vi "Test.vi"() -> ()   [LabVIEW 2022 SP3]
panel:
  out "error IO":errorcluster
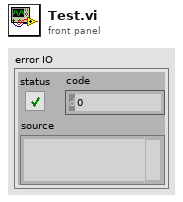
[diagram p1: front panel]
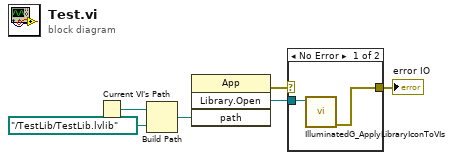
[diagram p0: block diagram]
diagram:
  n1 = Current VI's Path() -> (path=w5:path)
  n2 = Build Path(base path=w5, name or relative path=path "../TestLib/TestLib.lvlib") -> (appended path=w3:path)
  n3 = invoke class="App" method="Library.Open"("path"=w3) -> (error out=w2:errorcluster, "Open Library"=w6:refnum<vi>)  [unwired: 3 in, 2 out]
  n4 = case shown="No Error" w2 {
    selector: w2 -> [_ w9]
    tunnel: w6 -> [w8 _]
    tunnel: [w7 w9] -> w1
    frame No Error {
      n5 = call "IlluminatedG_ApplyLibraryIconToVIs.vi"("Library"=w8) -> ("error out"=w7:errorcluster)  [unwired: 10 in]
    }
    frame Error {
    }
  }
  "error IO" <- w1
